vi "VI Reentrancy.vi"(8 "error in (no error)":errorcluster, 11 "VI in":refnum<vi>) -> (0 "error out":errorcluster, 2 "Reentrancy":T1, 3 "VI":refnum<vi>)   [LabVIEW 2020, in "PropertyBinder.lvlib"]
uses:
  PropertyBinder.lvlib
  Reentrancy.ctl
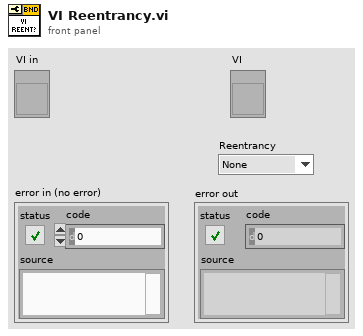
[diagram p1: front panel]
types:
  T1 = typedef "PropertyBinder.lvlib/Reentrancy.ctl" = enum16{"None", "Shared", "Preallocated"}
  T2 = enum16{"Share clones between instances", "Preallocate clone for each instance"}
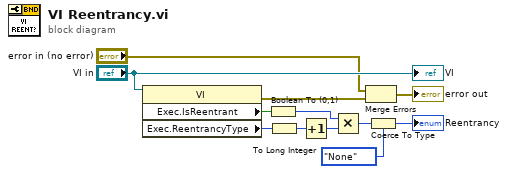
[diagram p0: block diagram]
diagram:
  n1 = property class="VI"(reference="VI in") -> (error out=w3:errorcluster, "Exec.IsReentrant"=w12:bool, "Exec.ReentrancyType"=w11:T2)  [unwired: 1 in, 1 out]
  n2 = Boolean To (0,1)(Boolean=w12) -> (0, 1=w9:i16)
  n3 = To Long Integer(number=w11) -> (32bit integer=w10:i32)
  n4 = Increment(x=w10) -> (x+1=w8:i32)
  n5 = Multiply(x=w9, y=w8) -> (x*y=w7:i32)
  n6 = Merge Errors("error in (no error)", w3) -> (→"error out":errorcluster)
  n7 = Coerce To Type(0:w7, 1:Reentrancy."None" ("Reentrancy")) -> (2:→"Reentrancy":T1)
  "VI" <- "VI in"
